vi "Iteration.vi"(11 "Plugin in":refnum<class "Plugin.lvclass">) -> (2 "Iteration":u64=1, 3 "Plugin out":refnum<class "Plugin.lvclass">)   [LabVIEW 2017, in "DSF Core.lvlib" / "Plugin.lvclass"]
uses:
  Plugin.lvclass
  Plugin.lvclass/Plugin.ctl
  Timing/Timing.lvclass/Timing.ctl
  Timing/Timing.lvclass
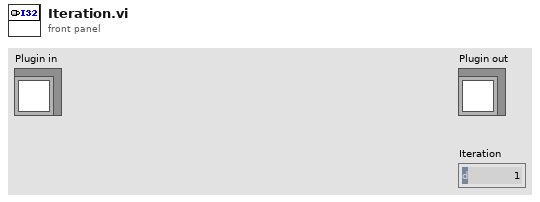
[diagram p1: front panel]
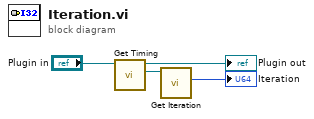
[diagram p0: block diagram]
diagram:
  n1 = call "Get Timing.vi"("Plugin in"="Plugin in") -> ("Timing"=w3:refnum<class "Timing.lvclass">, "Plugin out"=→"Plugin out":refnum<class "Plugin.lvclass">)  [unwired: 9 in]
  n2 = call "Get Iteration.vi"("Timing in"=w3) -> ("Iteration"=→"Iteration":u64)  [unwired: 9 in, 1 out]
